vi "Vector Field.vi"() -> ()   [LabVIEW 2013]
uses:
  <vilib>/Heliosphere Research LLC/Advanced Plotting Toolkit/api_core/NewPlotProperties.ctl
  <vilib>/Heliosphere Research LLC/Advanced Plotting Toolkit/typedefs/PlotColor.ctl
  <vilib>/Heliosphere Research LLC/Advanced Plotting Toolkit/api_plotting/VectorFieldProperties.ctl
  <vilib>/Heliosphere Research LLC/Advanced Plotting Toolkit/properties/Colormap.ctl
  <vilib>/Heliosphere Research LLC/Advanced Plotting Toolkit/properties/Colormap_Map.ctl
  <vilib>/Heliosphere Research LLC/Advanced Plotting Toolkit/properties/Colormap_Scaling.ctl
  <vilib>/Heliosphere Research LLC/Advanced Plotting Toolkit/properties/Display.ctl
  <vilib>/Heliosphere Research LLC/Advanced Plotting Toolkit/Advanced Plotting Toolkit.lvlib
panel:
  in  "Arrow Colors":T1(ring)=enum."X Vector Component"
  out "Vector Plot":picture
  # "Vector Field"
  # "This VI demonstrates the simplest way to visualize a vector\nfield: by plotting a field of arrows.\n\nA pair of 2D arrays are provided, one which gives the X\ncomponent at every point, and one which give the Y\ncomponent at every point.  The Toolkit then paints an arrow\nat each point of the appropriate size and direction.\n\nBy default, all the arrows will be colored black.  But if you\nsupply another 2D array to the Colormap Values input, its\nvalues will be used to color the arrows.\n\nThis demo shows the magnetic field around a wire of\nfinite size.  You can choose whether to color the arrows\naccording to the X or Y components, or the overall\nmagnitude of the vector at each point."
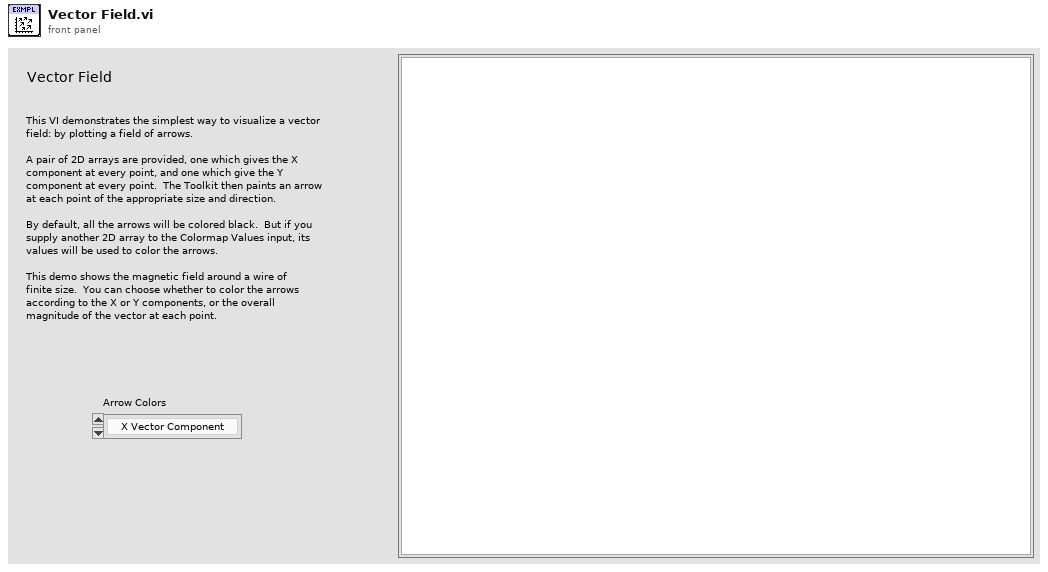
[diagram p1: front panel]
types:
  T1 = enum16{"Vector Magnitude", "X Vector Component", "Y Vector Component", "Plain Black"}
  T2 = typedef "Advanced Plotting Toolkit.lvlib/VectorFieldProperties.ctl" = cluster{"Color":T3, "Arrow Scale":dbl, "Colormap":T4, "Display":T7}
  T3 = typedef "Advanced Plotting Toolkit.lvlib/PlotColor.ctl" = u32
  T4 = typedef "Advanced Plotting Toolkit.lvlib/Colormap.ctl" = cluster{"Map":T5, "Value Min":dbl, "Value Max":dbl, "Scaling":T6, "Reverse":bool}
  T5 = typedef "Advanced Plotting Toolkit.lvlib/Colormap_Map.ctl" = enum16{"Automatic", "Rainbow", "Hot and Cold", "White-Black", "White-Blue", "White-Green", "White-Red", "Fire", "Water", "Earth", "Air", "Pastel", "Banded", "Stepped"}
  T6 = typedef "Advanced Plotting Toolkit.lvlib/Colormap_Scaling.ctl" = enum16{"Default"}
  T7 = typedef "Advanced Plotting Toolkit.lvlib/Display.ctl" = cluster{"Alpha":dbl, "Z Order":dbl}
  T8 = typedef "Advanced Plotting Toolkit.lvlib/NewPlotProperties.ctl" = cluster{"Background Color":T3, "Axis Background":T3, "Left Margin":dbl, "Right Margin":dbl, "Bottom Margin":dbl, "Top Margin":dbl, "Aspect Ratio":dbl}
  T9 = typedef "Advanced Plotting Toolkit.lvlib/PlotID.ctl" = i32
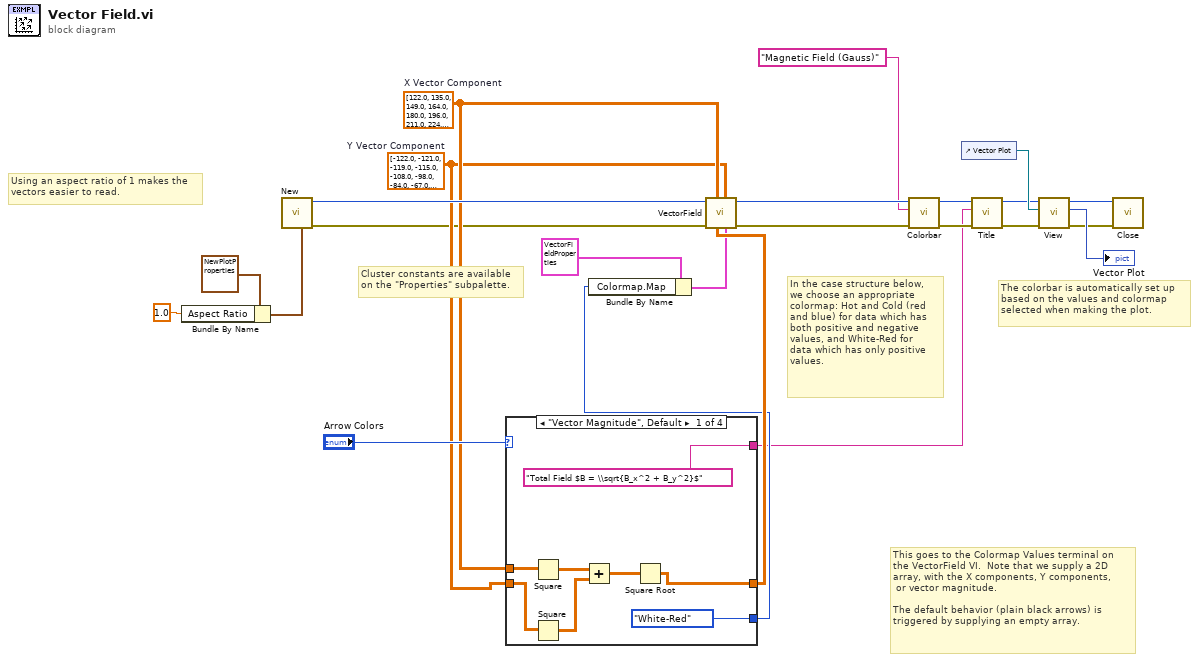
[diagram p0: block diagram]
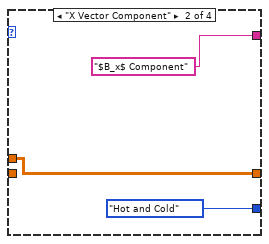
[diagram p2: hidden frame]
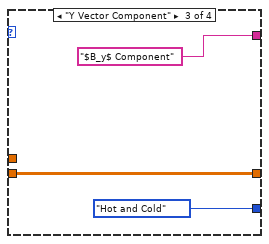
[diagram p3: hidden frame]
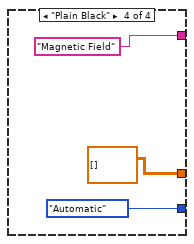
[diagram p4: hidden frame]
diagram:
  w14 = sgl[][] [[-122.0, -121.0, -119.0, -115.0, -108.0, -98.0, -84.0, -67.0, -47.0, -24.0, 0.0, 24.0, 47.0, 67.0, 84.0, 98.0, 108.0, 115.0, 119.0, 121.0], [-135.0, -136.0, -135.0, -131.0, -125.0, -115.0, -101.0, -81.0, -57.0, -29.0, 0.0, 29.0, 57.0, 81.0, 101.0, 115.0, 125.0, 131.0, 135.0, 136.0], [-149.0, -152.0, -153.0, -151.0, -147.0, -137.0, -122.0, -100.0, -72.0, -37.0, 0.0, 37.0, 72.0, 100.0, 122.0, 137.0, 147.0, 151.0, 153.0, 152.0], [-164.0, -169.0, -173.0, -175.0, -172.0, -165.0, -150.0, -126.0, -92.0, -49.0, 0.0, 49.0, 92.0, 126.0, 150.0, 165.0, 172.0, 175.0, 173.0, 169.0], [-180.0, -188.0, -196.0, -201.0, -204.0, -200.0, -188.0, -150.0, -100.0, -50.0, 0.0, 50.0, 100.0, 150.0, 188.0, 200.0, 204.0, 201.0, 196.0, 188.0], [-196.0, -208.0, -220.0, -231.0, -240.0, -245.0, -200.0, -150.0, -100.0, -50.0, 0.0, 50.0, 100.0, 150.0, 200.0, 245.0, 240.0, 231.0, 220.0, 208.0], [-211.0, -227.0, -245.0, -263.0, -282.0, -250.0, -200.0, -150.0, -100.0, -50.0, 0.0, 50.0, 100.0, 150.0, 200.0, 250.0, 282.0, 263.0, 245.0, 227.0], [-224.0, -245.0, -268.0, -295.0, -300.0, -250.0, -200.0, -150.0, -100.0, -50.0, 0.0, 50.0, 100.0, 150.0, 200.0, 250.0, 300.0, 295.0, 268.0, 245.0], [-235.0, -259.0, -288.0, -323.0, -300.0, -250.0, -200.0, -150.0, -100.0, -50.0, 0.0, 50.0, 100.0, 150.0, 200.0, 250.0, 300.0, 323.0, 288.0, 259.0], [-242.0, -268.0, -301.0, -343.0, -300.0, -250.0, -200.0, -150.0, -100.0, -50.0, 0.0, 50.0, 100.0, 150.0, 200.0, 250.0, 300.0, 343.0, 301.0, 268.0], [-245.0, -272.0, -306.0, -350.0, -300.0, -250.0, -200.0, -150.0, -100.0, -50.0, 0.0, 50.0, 100.0, 150.0, 200.0, 250.0, 300.0, 350.0, 306.0, 272.0], [-242.0, -268.0, -301.0, -343.0, -300.0, -250.0, -200.0, -150.0, -100.0, -50.0, 0.0, 50.0, 100.0, 150.0, 200.0, 250.0, 300.0, 343.0, 301.0, 268.0], [-235.0, -259.0, -288.0, -323.0, -300.0, -250.0, -200.0, -150.0, -100.0, -50.0, 0.0, 50.0, 100.0, 150.0, 200.0, 250.0, 300.0, 323.0, 288.0, 259.0], [-224.0, -245.0, -268.0, -295.0, -300.0, -250.0, -200.0, -150.0, -100.0, -50.0, 0.0, 50.0, 100.0, 150.0, 200.0, 250.0, 300.0, 295.0, 268.0, 245.0], [-211.0, -227.0, -245.0, -263.0, -282.0, -250.0, -200.0, -150.0, -100.0, -50.0, 0.0, 50.0, 100.0, 150.0, 200.0, 250.0, 282.0, 263.0, 245.0, 227.0], [-196.0, -208.0, -220.0, -231.0, -240.0, -245.0, -200.0, -150.0, -100.0, -50.0, 0.0, 50.0, 100.0, 150.0, 200.0, 245.0, 240.0, 231.0, 220.0, 208.0], [-180.0, -188.0, -196.0, -201.0, -204.0, -200.0, -188.0, -150.0, -100.0, -50.0, 0.0, 50.0, 100.0, 150.0, 188.0, 200.0, 204.0, 201.0, 196.0, 188.0], [-164.0, -169.0, -173.0, -175.0, -172.0, -165.0, -150.0, -126.0, -92.0, -49.0, 0.0, 49.0, 92.0, 126.0, 150.0, 165.0, 172.0, 175.0, 173.0, 169.0], [-149.0, -152.0, -153.0, -151.0, -147.0, -137.0, -122.0, -100.0, -72.0, -37.0, 0.0, 37.0, 72.0, 100.0, 122.0, 137.0, 147.0, 151.0, 153.0, 152.0], [-135.0, -136.0, -135.0, -131.0, -125.0, -115.0, -101.0, -81.0, -57.0, -29.0, 0.0, 29.0, 57.0, 81.0, 101.0, 115.0, 125.0, 131.0, 135.0, 136.0]]  # Y Vector Component
  w15 = sgl[][] [[122.0, 135.0, 149.0, 164.0, 180.0, 196.0, 211.0, 224.0, 235.0, 242.0, 245.0, 242.0, 235.0, 224.0, 211.0, 196.0, 180.0, 164.0, 149.0, 135.0], [121.0, 136.0, 152.0, 169.0, 188.0, 208.0, 227.0, 245.0, 259.0, 268.0, 272.0, 268.0, 259.0, 245.0, 227.0, 208.0, 188.0, 169.0, 152.0, 136.0], [119.0, 135.0, 153.0, 173.0, 196.0, 220.0, 245.0, 268.0, 288.0, 301.0, 306.0, 301.0, 288.0, 268.0, 245.0, 220.0, 196.0, 173.0, 153.0, 135.0], [115.0, 131.0, 151.0, 175.0, 201.0, 231.0, 263.0, 295.0, 323.0, 343.0, 350.0, 343.0, 323.0, 295.0, 263.0, 231.0, 201.0, 175.0, 151.0, 131.0], [108.0, 125.0, 147.0, 172.0, 204.0, 240.0, 282.0, 300.0, 300.0, 300.0, 300.0, 300.0, 300.0, 300.0, 282.0, 240.0, 204.0, 172.0, 147.0, 125.0], [98.0, 115.0, 137.0, 165.0, 200.0, 245.0, 250.0, 250.0, 250.0, 250.0, 250.0, 250.0, 250.0, 250.0, 250.0, 245.0, 200.0, 165.0, 137.0, 115.0], [84.0, 101.0, 122.0, 150.0, 188.0, 200.0, 200.0, 200.0, 200.0, 200.0, 200.0, 200.0, 200.0, 200.0, 200.0, 200.0, 188.0, 150.0, 122.0, 101.0], [67.0, 81.0, 100.0, 126.0, 150.0, 150.0, 150.0, 150.0, 150.0, 150.0, 150.0, 150.0, 150.0, 150.0, 150.0, 150.0, 150.0, 126.0, 100.0, 81.0], [47.0, 57.0, 72.0, 92.0, 100.0, 100.0, 100.0, 100.0, 100.0, 100.0, 100.0, 100.0, 100.0, 100.0, 100.0, 100.0, 100.0, 92.0, 72.0, 57.0], [24.0, 29.0, 37.0, 49.0, 50.0, 50.0, 50.0, 50.0, 50.0, 50.0, 50.0, 50.0, 50.0, 50.0, 50.0, 50.0, 50.0, 49.0, 37.0, 29.0], [0.0, 0.0, 0.0, 0.0, 0.0, 0.0, 0.0, 0.0, 0.0, 0.0, 0.0, 0.0, 0.0, 0.0, 0.0, 0.0, 0.0, 0.0, 0.0, 0.0], [-24.0, -29.0, -37.0, -49.0, -50.0, -50.0, -50.0, -50.0, -50.0, -50.0, -50.0, -50.0, -50.0, -50.0, -50.0, -50.0, -50.0, -49.0, -37.0, -29.0], [-47.0, -57.0, -72.0, -92.0, -100.0, -100.0, -100.0, -100.0, -100.0, -100.0, -100.0, -100.0, -100.0, -100.0, -100.0, -100.0, -100.0, -92.0, -72.0, -57.0], [-67.0, -81.0, -100.0, -126.0, -150.0, -150.0, -150.0, -150.0, -150.0, -150.0, -150.0, -150.0, -150.0, -150.0, -150.0, -150.0, -150.0, -126.0, -100.0, -81.0], [-84.0, -101.0, -122.0, -150.0, -188.0, -200.0, -200.0, -200.0, -200.0, -200.0, -200.0, -200.0, -200.0, -200.0, -200.0, -200.0, -188.0, -150.0, -122.0, -101.0], [-98.0, -115.0, -137.0, -165.0, -200.0, -245.0, -250.0, -250.0, -250.0, -250.0, -250.0, -250.0, -250.0, -250.0, -250.0, -245.0, -200.0, -165.0, -137.0, -115.0], [-108.0, -125.0, -147.0, -172.0, -204.0, -240.0, -282.0, -300.0, -300.0, -300.0, -300.0, -300.0, -300.0, -300.0, -282.0, -240.0, -204.0, -172.0, -147.0, -125.0], [-115.0, -131.0, -151.0, -175.0, -201.0, -231.0, -263.0, -295.0, -323.0, -343.0, -350.0, -343.0, -323.0, -295.0, -263.0, -231.0, -201.0, -175.0, -151.0, -131.0], [-119.0, -135.0, -153.0, -173.0, -196.0, -220.0, -245.0, -268.0, -288.0, -301.0, -306.0, -301.0, -288.0, -268.0, -245.0, -220.0, -196.0, -173.0, -153.0, -135.0], [-121.0, -136.0, -152.0, -169.0, -188.0, -208.0, -227.0, -245.0, -259.0, -268.0, -272.0, -268.0, -259.0, -245.0, -227.0, -208.0, -188.0, -169.0, -152.0, -136.0]]  # X Vector Component
  # "Cluster constants are available\non the \"Properties\" subpalette."
  # "In the case structure below,\nwe choose an appropriate\ncolormap: Hot and Cold (red\nand blue) for data which has\nboth positive and negative\nvalues, and White-Red for\ndata which has only positive\nvalues."
  # "The colorbar is automatically set up\nbased on the values and colormap \nselected when making the plot."
  # "This goes to the Colormap Values terminal on\nthe VectorField VI.  Note that we supply a 2D\narray, with the X components, Y components,\n or vector magnitude.\n\nThe default behavior (plain black arrows) is\ntriggered by supplying an empty array."
  # "Using an aspect ratio of 1 makes the\nvectors easier to read."
  n1 = Bundle By Name(cluster=T8 {"Background Color"=2147483647, "Axis Background"=2147483647, "Left Margin"=nan, "Right Margin"=nan, "Bottom Margin"=nan, "Top Margin"=nan, "Aspect Ratio"=nan} ("New Plot Properties"), "Aspect Ratio"=1.0) -> (w16:T8)
  n2 = call <vilib>:"New.vi"("Properties"=w16) -> ("error out"=w12:errorcluster, "Plot ID"=w21:T9)  [unwired: 9 in]
  n3 = case shown="\"Vector Magnitude\", Default" "Arrow Colors" {
    tunnel: w15 -> [w32 w35 _ _]
    tunnel: w14 -> [w31 _ w38 _]
    tunnel: [w27 w35 w38 sgl[][] [] ("Y Vector Component")] -> w13
    tunnel: [Colormap_Map."White-Red" ("Colormap.Map") Colormap_Map."Hot and Cold" ("Colormap.Map") Colormap_Map."Hot and Cold" ("Colormap.Map") Colormap_Map."Automatic" ("Colormap.Map")] -> w9
    tunnel: ["Total Field $B = \\sqrt{B_x^2 + B_y^2}$" "$B_x$ Component" "$B_y$ Component" "Magnetic Field"] -> w3
    frame "Vector Magnitude", Default {
      n4 = Square(x=w32) -> (x^2=w30:sgl[][])
      n5 = Square(x=w31) -> (x^2=w29:sgl[][])
      n6 = Add(x=w30, y=w29) -> (x+y=w28:sgl[][])
      n7 = Square Root(x=w28) -> (sqrt(x)=w27:sgl[][])
    }
    frame "X Vector Component" {
    }
    frame "Y Vector Component" {
    }
    frame "Plain Black" {
    }
  }
  n8 = Bundle By Name(cluster=T2 {"Color"=2147483647, "Arrow Scale"=nan, "Colormap"={"Map"=enum."Automatic", "Value Min"=nan, "Value Max"=nan, "Scaling"=enum."Default", "Reverse"=FALSE}, "Display"={"Alpha"=nan, "Z Order"=nan}} ("Vector Field Properties"), "Colormap.Map"=w9) -> (w8:T2)
  n9 = call <vilib>:"VectorField.vi"("Properties"=w8, "Y Vector Component"=w14, "Colormap Values"=w13, "X Vector Component"=w15, "error in (no error)"=w12, "Plot ID"=w21) -> ("error out"=w11:errorcluster, "Plot ID Out"=w19:T9)  [unwired: 4 in]
  n10 = call <vilib>:"Colorbar.vi"("error in (no error)"=w11, "Label"="Magnetic Field (Gauss)", "Plot ID"=w19) -> ("error out"=w6:errorcluster, "Plot ID Out"=w7:T9)  [unwired: 7 in]
  n11 = control-ref of="Vector Plot"() -> (w23:refnum<vi>)
  n12 = call <vilib>:"Title.vi"("error in (no error)"=w6, "Title"=w3, "Plot ID"=w7) -> ("error out"=w4:errorcluster, "Plot ID out"=w5:T9)  [unwired: 7 in]
  n13 = call <vilib>:"View.vi"("error in (no error)"=w4, "Ref for Sizing"=w23, "Plot ID"=w5) -> ("error out"=w1:errorcluster, "Picture"=→"Vector Plot":picture, "Plot ID Out"=w22:T9)  [unwired: 6 in]
  n14 = call <vilib>:"Close.vi"("error in (no error)"=w1, "Plot ID"=w22) -> ()  [unwired: 9 in, 1 out]
